vi "Iterate.vi"(0 "Initial Error":dbl=0.01 min=-1000000000.0 max=1000000000.0 format="%.2f", 1 "Initial Pullability":dbl format="%.6f", 2 "Gate Time":T1(ring)=enum."1.0 second", 4 "V_inject Initial":dbl format="%.6f", 5 "Tolerence":dbl format="%.2f", 6 "Frequency":dbl format="%.2f", 7 "V Low Limit":dbl format="%.4f", 10 "Frequency Channel":enum16{"Channel 1", "Channel 2", "Channel 3"}(ring), 11 "Frequency Address":u8=30 max=31 step=1, 12 "V High Limit":dbl format="%.4f", 13 "Power Supply Address":u8=5, 16 "PowerSupplyType":i32, 17 "Output Terminals(+6 V:0)":u16(ring) items=["+6 V output", "+25 V output", "-25 V output"]) -> (9 "Measured Frequency":dbl[](array[numeric]) format="%.6f", 14 "Pullability":dbl[](array[numeric]) format="%.6f", 15 "Error":dbl[](array[numeric]) format="%.2f", 18 "Iteration Successful":bool[](array[boolean]), 19 "V_inject":dbl[](array[numeric]) format="%.6f")   [LabVIEW 2024]
panel:
  # "INPUT PARAMETERS"
  # "OUTPUT DATA"
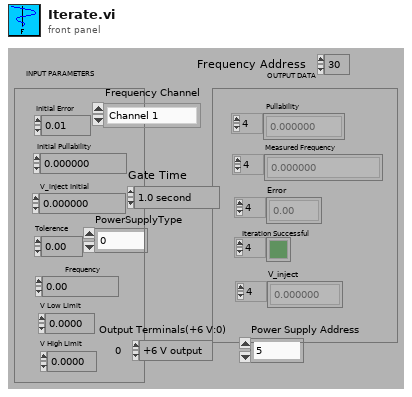
[diagram p1: front panel]
types:
  T1 = enum16{"0.1 second", "1.0 second", "10.0 second"}
  T2 = cluster{"error":bool, "code":i32, "source":string}
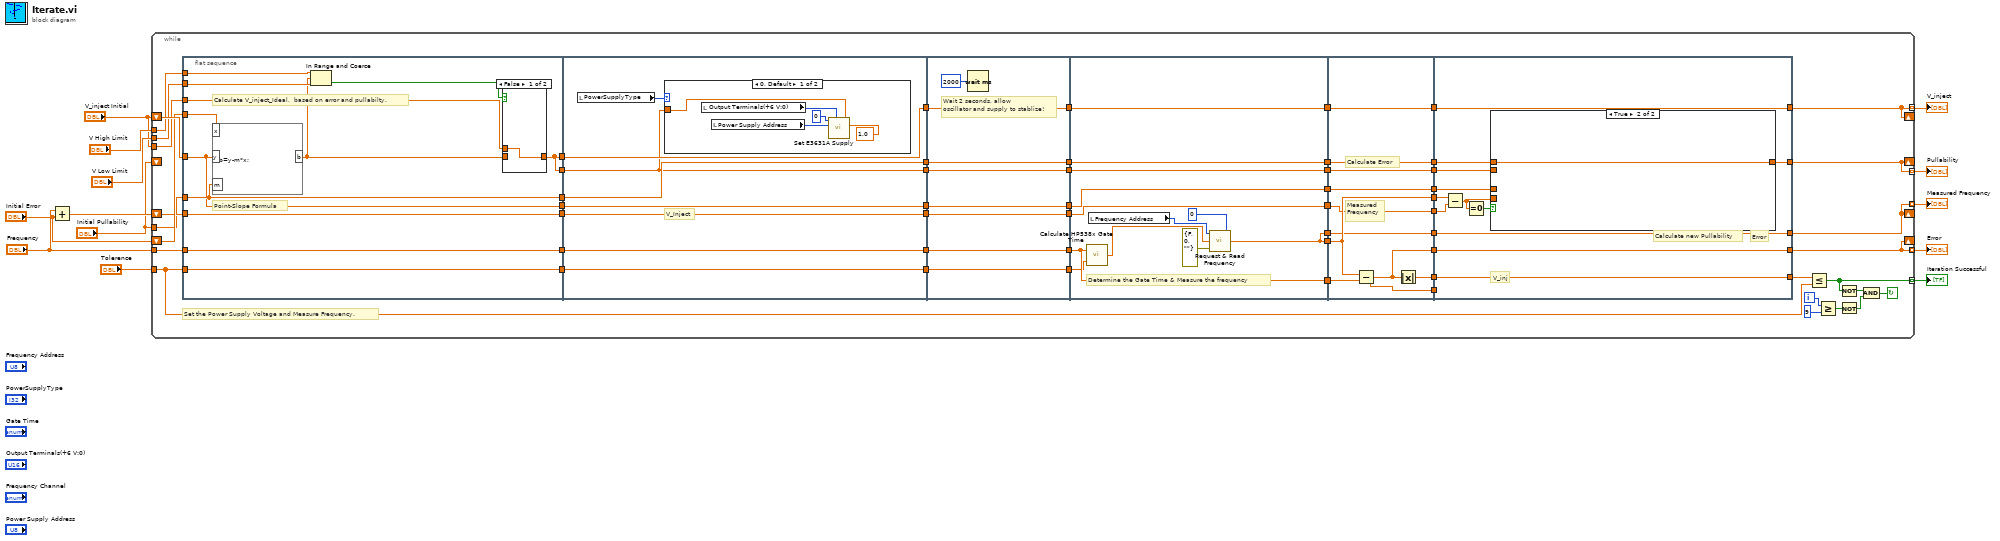
[diagram p0: block diagram]
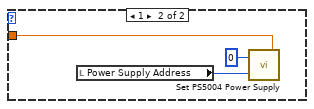
[diagram p3: hidden frame]
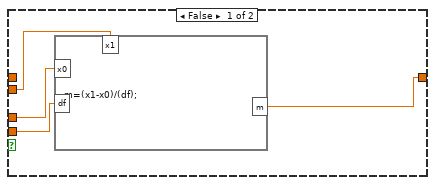
[diagram p4: hidden frame]
diagram:
  n1 = Add(x="Frequency", y="Initial Error") -> (x+y=w5:dbl)
  n2 = while {
    tunnel: "Tolerence" -> [w56]
    tunnel: [w67] -> w12 mode=indexing
    shift-right: [w62] -> _
    shift-left: "V_inject Initial" -> [w66]
    shift-right: [w63] -> _
    shift-left: "Initial Error" -> [w65]
    tunnel: [w60] -> w11 mode=indexing
    tunnel: "Frequency" -> [w64]
    tunnel: [w63] -> w8 mode=indexing
    tunnel: [w62] -> w7 mode=indexing
    tunnel: [w59] -> w6 mode=indexing
    shift-right: [w60] -> _
    shift-left: w5 -> [w61]
    shift-right: [w59] -> _
    shift-left: "Initial Pullability" -> [_]
    tunnel: "Initial Pullability" -> [w57]
    tunnel: "V Low Limit" -> [w54]
    tunnel: "V High Limit" -> [w55]
    tunnel: "V_inject Initial" -> [w53]
    i -> [w58]
    stop <- w71 continue-if-true
    # "Set the Power Supply Voltage and Measure Frequency."
    n3 = flat-sequence {
      tunnel: w65 -> [w83]
      tunnel: w57 -> [w85]
      tunnel: [w85] -> w52
      tunnel: w66 -> [w84]
      tunnel: [w84] -> w51
      tunnel: w64 -> [w76]
      tunnel: [w76] -> w50
      tunnel: [w79] -> w49
      tunnel: w61 -> [w75]
      tunnel: [w75] -> w48
      tunnel: w56 -> [w74]
      tunnel: [w74] -> w47
      tunnel: w55 -> [w81]
      tunnel: w54 -> [w82]
      tunnel: w53 -> [w77]
      tunnel: [w79] -> w46
      tunnel: w52 -> [w95]
      tunnel: [w95] -> w45
      tunnel: w51 -> [w94]
      tunnel: [w94] -> w44
      tunnel: w50 -> [w93]
      tunnel: [w93] -> w43
      tunnel: w49 -> [w92]
      tunnel: [w92] -> w42
      tunnel: w48 -> [w91]
      tunnel: [w91] -> w41
      tunnel: w47 -> [w90]
      tunnel: [w90] -> w40
      tunnel: w46 -> [w89]
      tunnel: [w89] -> w39
      tunnel: w45 -> [w110]
      tunnel: [w110] -> w38
      tunnel: w44 -> [w109]
      tunnel: [w109] -> w37
      tunnel: w43 -> [w108]
      tunnel: [w108] -> w36
      tunnel: w42 -> [w107]
      tunnel: [w107] -> w35
      tunnel: w41 -> [w106]
      tunnel: [w106] -> w34
      tunnel: w40 -> [w105]
      tunnel: [w105] -> w33
      tunnel: w39 -> [w104]
      tunnel: [w104] -> w32
      tunnel: w38 -> [w121]
      tunnel: [w121] -> w31
      tunnel: w37 -> [w120]
      tunnel: [w120] -> w30
      tunnel: [w116] -> w29
      tunnel: w36 -> [w123]
      tunnel: [w123] -> w28
      tunnel: w35 -> [w119]
      tunnel: [w119] -> w27
      tunnel: w34 -> [w118]
      tunnel: [w118] -> w26
      tunnel: w33 -> [w122]
      tunnel: [w116] -> w25
      tunnel: w32 -> [w117]
      tunnel: [w117] -> w24
      tunnel: [w133] -> w23
      tunnel: [w132] -> w22
      tunnel: w31 -> [w129]
      tunnel: [w129] -> w21
      tunnel: w30 -> [w128]
      tunnel: [w128] -> w20
      tunnel: w29 -> [w127]
      tunnel: [w127] -> w19
      tunnel: w28 -> [w130]
      tunnel: w27 -> [w126]
      tunnel: [w126] -> w18
      tunnel: w26 -> [w125]
      tunnel: [w125] -> w17
      tunnel: w25 -> [w131]
      tunnel: [w131] -> w16
      tunnel: w24 -> [w124]
      tunnel: [w124] -> w15
      tunnel: [w132] -> w14
      tunnel: [w143] -> w73
      tunnel: [w142] -> w63
      tunnel: [w141] -> w60
      tunnel: [w140] -> w62
      tunnel: [w139] -> w59
      tunnel: w14 -> [_]
      tunnel: w15 -> [w145]
      tunnel: w16 -> [w144]
      tunnel: w17 -> [w134]
      tunnel: w18 -> [w140]
      tunnel: w19 -> [w141]
      tunnel: w20 -> [w136]
      tunnel: w21 -> [w137]
      tunnel: w22 -> [w142]
      tunnel: w23 -> [w143]
      frame #0 {
        # "Calculate V_inject_Ideal,  based on error and pullabilty."
        # "Point-Slope Formula"
        n4 = formula code="b=y-m*x;"("y"=w84, "m"=w85, "x"=w83) -> ("b"=w78:dbl)
        n5 = In Range and Coerce(upper limit=w81, x=w78, lower limit=w82) -> (In Range?=w80:bool)  [unwired: 1 out]
        n6 = case shown="False" w80 {
          tunnel: [w86 w87] -> w79
          tunnel: w78 -> [_ w87]
          tunnel: w77 -> [w86 _]
          frame False {
          }
          frame True {
          }
        }
      }
      frame #1 {
        # "V_Inject"
        n7 = local read "PowerSupplyType"() -> (w88:i32)
        n8 = case shown="0, Default" w88 {
          tunnel: w89 -> [w100 w102]
          frame 0, Default {
            n9 = local read "Output Terminals(+6 V:0)"() -> (w97:u16)
            n10 = local read "Power Supply Address"() -> (w98:u8)
            n11 = call "Set E3631A Supply.vi"("Current Limit"=1.0, "Voltage Limit"=w100, "Output Terminals(+6 V:0)"=w97, "Address"=w98, "GPIB#"=u8 0) -> ()  [unwired: 3 in, 1 out]
          }
          frame 1 {
            n12 = local read "Power Supply Address"() -> (w101:u8)
            n13 = call "Set PS5004 Power Supply.vi"("Voltage"=w102, "Address"=w101, "System#"=0) -> ()
          }
        }
      }
      frame #2 {
        # "Wait 2 seconds, allow \noscillator and supply to stablize!"
        n14 = Wait (ms)(milliseconds to wait=u32 2000) -> ()  [unwired: 1 out]
      }
      frame #3 {
        # "Determine the Gate Time & Measure the frequency"
        n15 = call "Calculate HP538x Gate Time.vi"("Tolerence"=w122, "Nominal Frequency"=w123) -> ("Gate Time(Seconds)"=w115:dbl)
        n16 = local read "Frequency Address"() -> (w112:u8)
        n17 = call "Request & Read Frequency.vi"("System#"=u8 0, "error in"=T2 {"error"=FALSE, "code"=0, "source"=""}, "Gate Time"=w115, "GPIB Address"=w112) -> ("Measured Frequency"=w116:dbl)  [unwired: 1 out]
      }
      frame #4 {
        # "Measured\nFrequency"
        # "Calculate Error"
        n18 = Subtract(x=w131, y=w130) -> (x-y=w132:dbl)
        n19 = Absolute Value(x=w132) -> (abs(x)=w133:dbl)
      }
      frame #5 {
        # "V_inj"
        # "Error"
        # "Calculate new Pullability"
        n20 = Subtract(x=w144, y=w134) -> (x-y=w135:dbl)
        n21 = Equal To 0?(x=w135) -> (x = 0?=w138:bool)
        n22 = case shown="True" w138 {
          tunnel: [w149 w150] -> w139
          tunnel: w137 -> [_ w150]
          tunnel: w136 -> [w146 _]
          tunnel: w145 -> [w147 _]
          tunnel: w135 -> [w148 _]
          frame False {
            n23 = formula code="m=(x1-x0)/(df);"("x0"=w146, "x1"=w147, "df"=w148) -> ("m"=w149:dbl)
          }
          frame True {
          }
        }
      }
    }
    n24 = Less Or Equal?(x=w73, y=w56) -> (x <= y?=w67:bool)
    n25 = Greater Or Equal?(x=w58, y=9) -> (x >= y?=w70:bool)
    n26 = Not(x=w67) -> (.not. x?=w68:bool)
    n27 = Not(x=w70) -> (.not. x?=w69:bool)
    n28 = And(x=w68, y=w69) -> (x .and. y?=w71:bool)
  }
  "Iteration Successful" <- w12
  "Error" <- w8
  "Measured Frequency" <- w11
  "Pullability" <- w6
  "V_inject" <- w7
